vi "Convert 1D to 2D Double.vi"(9 "size(s)":i32[](array[numeric]), 11 "1D Array":dbl[](array[numeric])) -> (3 "2D Array":dbl[][](array[numeric]))   [LabVIEW 2014]
doc: "<B>Copyright</B>: (c) MHWirth 2015. All rights are reserved.\n\nThis subVI reshapes the input 1D array to 2D array based on the given sizes."
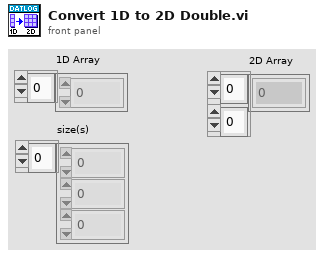
[diagram p1: front panel]
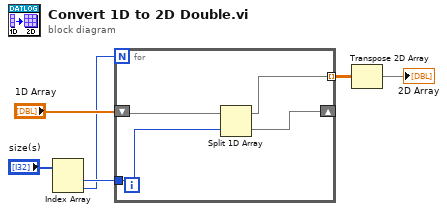
[diagram p0: block diagram]
diagram:
  n1 = Index Array(array="size(s)") -> (element #1=w4:i32, element #2=w3:i32)  [unwired: 2 in]
  n2 = for {
    N: w3 -> [_]
    tunnel: w4 -> [w9]
    tunnel: [w8] -> w2 mode=indexing
    shift-right: [w7] -> _
    shift-left: "1D Array" -> [w10]
    n3 = Split 1D Array(array=w10, index=w9) -> (first subarray=w8:dbl[], second subarray=w7:dbl[])
  }
  n4 = Transpose 2D Array(2D array=w2) -> (transposed array=→"2D Array":dbl[][])
